vi "Render Empty List Section.vi"(8 "Error In":errorcluster) -> (0 "Error Out":errorcluster)   [LabVIEW 2018, in "Tests.lvlib" / "Render.lvlib"]
uses:
  Render.lvlib
  src/Toolkit/Data/Array/Array.lvclass
  D:/Users/cfield/Code/Field R&D Services/Labstache/src/Toolkit/Data/Datum/Datum.lvclass
  src/Toolkit/Data/Map/Map.lvclass
  src/Toolkit/Data/Array/Support/From Strings.vi
  src/Toolkit/Data/Map/Support/From Datum.vi
  src/Toolkit/Low-Level/Renderer/Renderer.lvclass
  <vilib>/addons/_JKI Toolkits/Caraya/classes/Test/Test.lvclass
  <vilib>/addons/_JKI Toolkits/Caraya/classes/Assert/Assert.lvclass
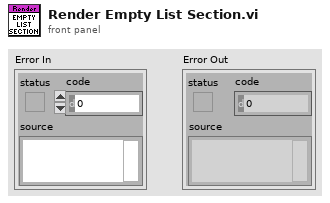
[diagram p1: front panel]
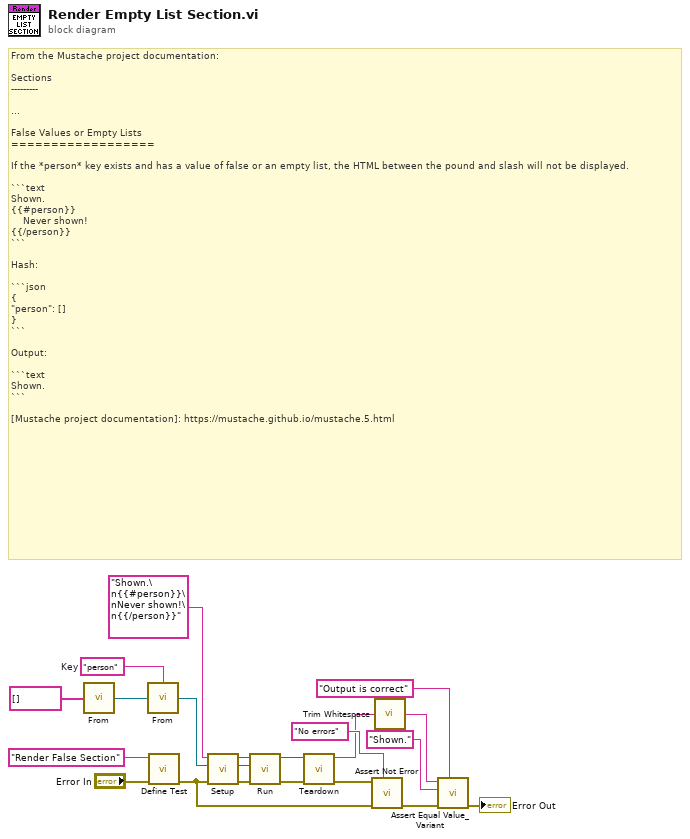
[diagram p0: block diagram]
diagram:
  w11 = "person"  # Key
  # "From the Mustache project documentation:\n\nSections\n---------\n\n...\n\nFalse Values or Empty Lists\n==================\n\nIf the *person* key exists and has a value of false or an empty list, the HTML between the pound and slash will not be displayed.\n\n```text\nShown.\n{{#person}}\n    Never shown!\n{{/person}}\n```\n\nHash:\n\n```json\n{\n\"person\": []\n}\n```\n\nOutput:\n\n```text\nShown.\n```\n\n[Mustache project documentation]: https://mustache.github.io/mustache.5.html"
  n1 = call-poly "From.vi"("Strings"=string[] []) -> ("Array"=w5:refnum<class "Array.lvclass">)  [unwired: 1 in]
  n2 = call-poly "From.vi"("Value"=w5, "Key"=w11) -> ("Map"=w3:refnum<class "Map.lvclass">)
  n3 = call <vilib>:"Define Test.vi"("error in (no error)"="Error In", "Label (VI Title)"="Render False Section") -> ("error out"=w8:errorcluster)  [unwired: 9 in]
  n4 = call "Setup.vi"("Error In"=w8, "Data"=w3, "Value"="Shown.\n{{#person}}\nNever shown!\n{{/person}}" ("format string")) -> ("Error Out"=w12:errorcluster, "Abstract Syntax Tree"=w2:refnum<class "Root.lvclass">, "Renderer"=w13:refnum<class "Renderer.lvclass">)  [unwired: 6 in]
  n5 = call-dynamic "Run.vi"("Error In"=w12, "Abstract Syntax Tree"=w2, "Renderer In"=w13) -> ("Error Out"=w14:errorcluster, "Renderer Out"=w1:refnum<class "Renderer.lvclass">)  [unwired: 7 in]
  n6 = call "Teardown.vi"("Error In"=w14, "Renderer"=w1) -> ("Error Out"=w15:errorcluster, "Output"=w7:string)  [unwired: 8 in]
  n7 = call <vilib>:"Assert Not Error.vi"("Label"="No errors", "error in (no error)"=w8, "Not Error?"=w15) -> ("error out"=w18:errorcluster)  [unwired: 8 in]
  n8 = call <vilib>:"Trim Whitespace.vi"("string"=w7) -> ("trimmed string"=w6:string)  [unwired: 1 in]
  n9 = call <vilib>:"Assert Equal Value_Variant.vi"("Label"="Output is correct", "error in (no error)"=w18, "Y"="Shown." ("Output"), "X"=w6) -> ("error out"=→"Error Out":errorcluster)  [unwired: 7 in]
